vi "credentialCheck.vi"(0 "connection ID in":refnum<k5>, 1 "error in":errorcluster) -> (2 "connection ID out":refnum<k5>, 3 "user":string, 4 "error out":errorcluster)   [LabVIEW 2011]
panel:
  out "Error Parm":errorcluster
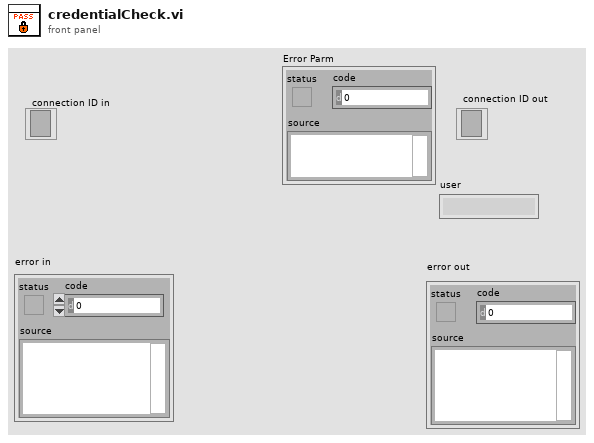
[diagram p1: front panel]
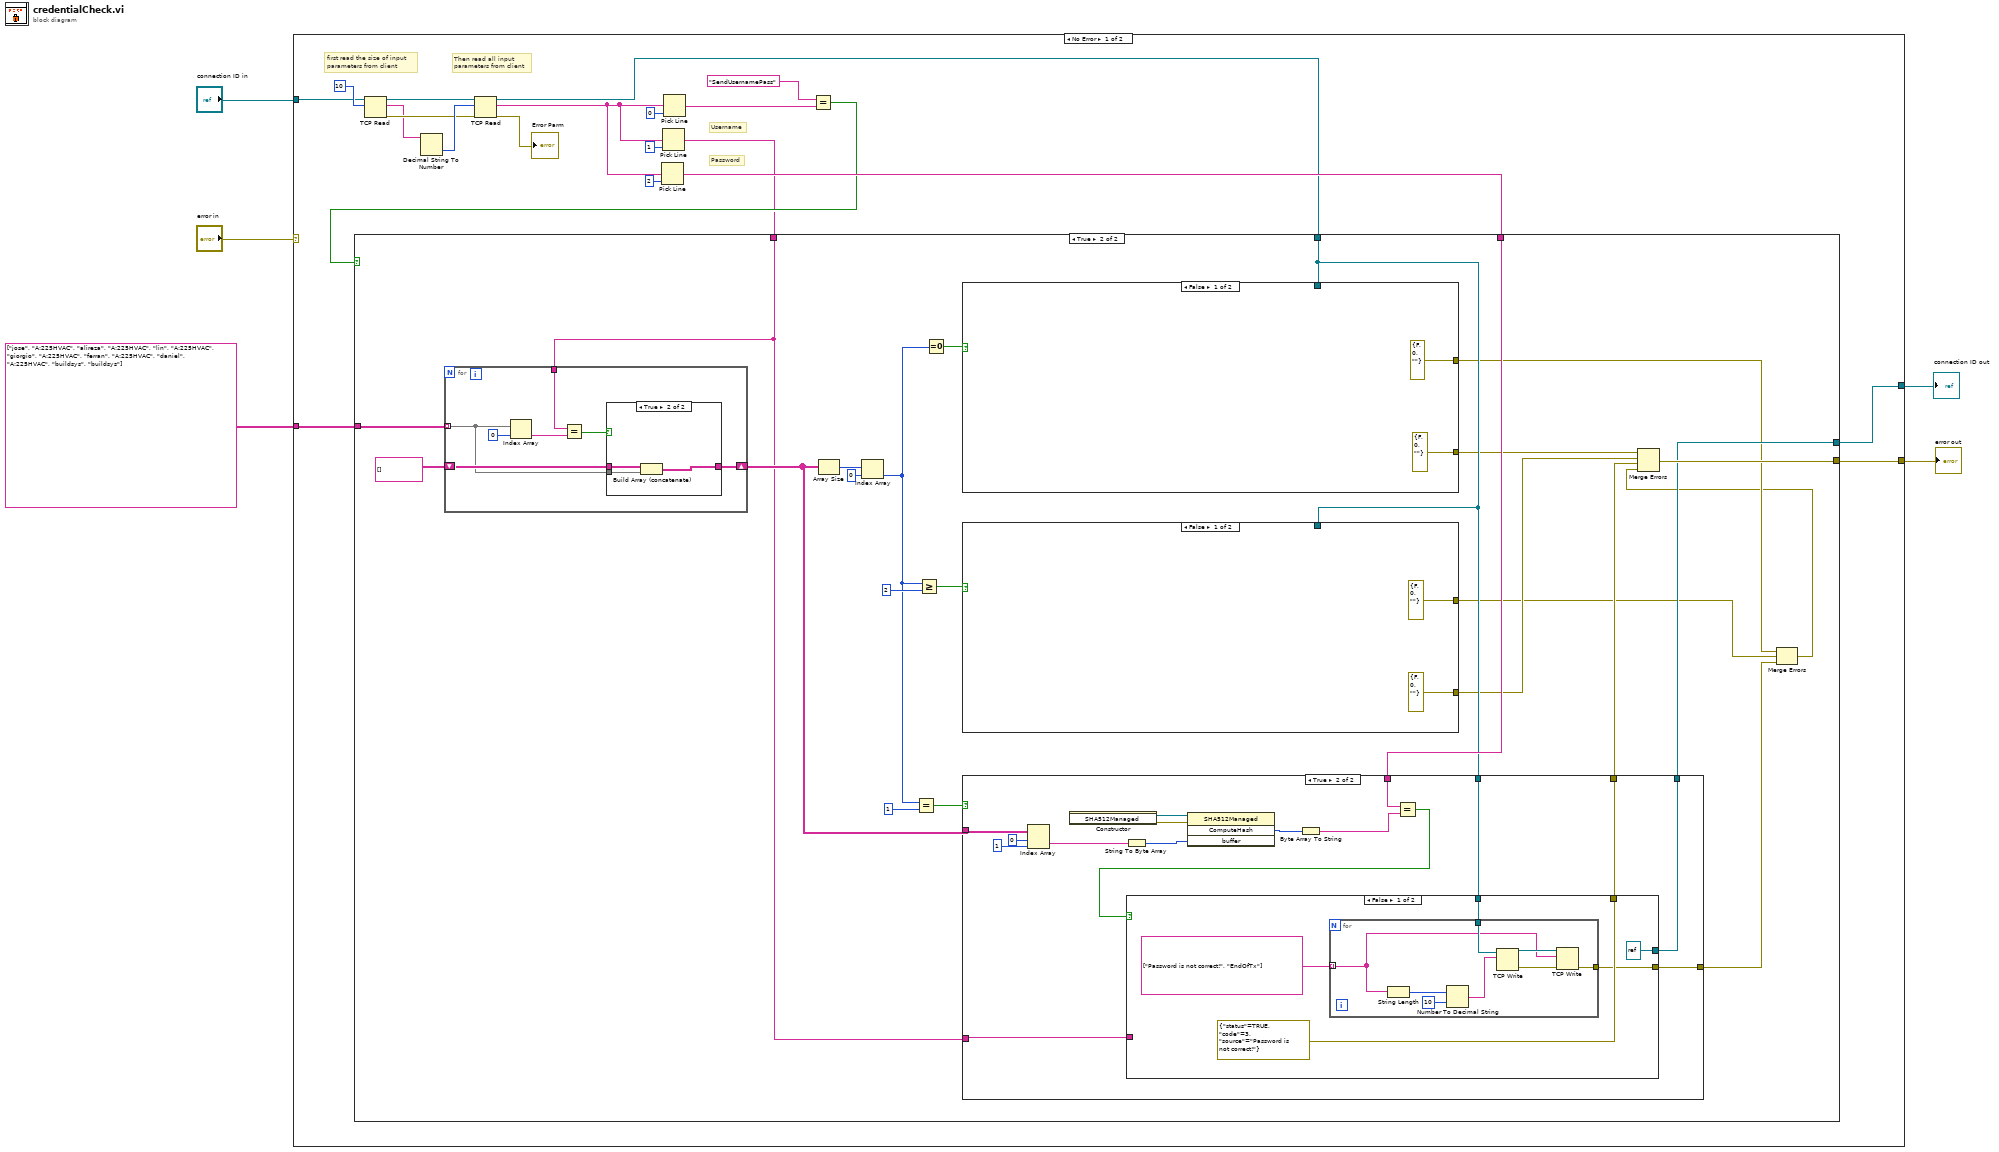
[diagram p0: block diagram]
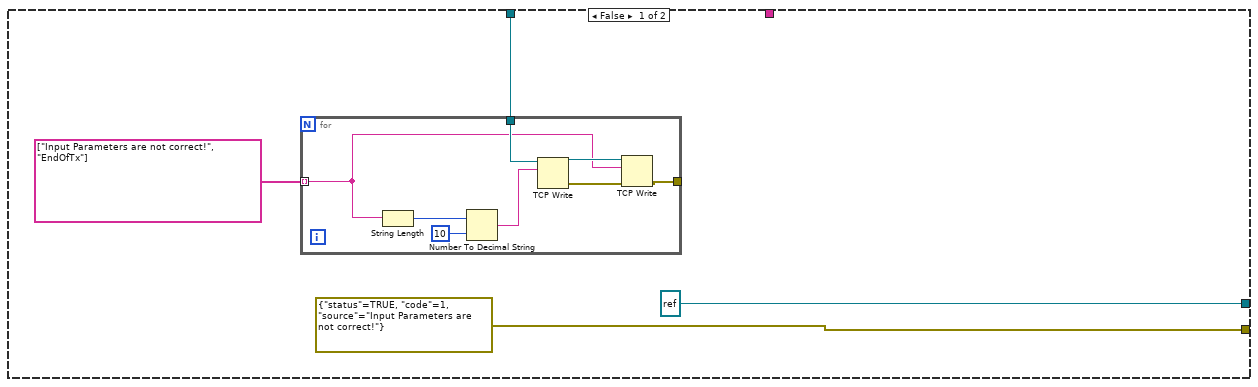
[diagram p2: hidden frame]
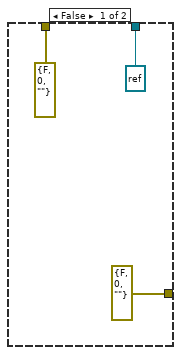
[diagram p3: hidden frame]
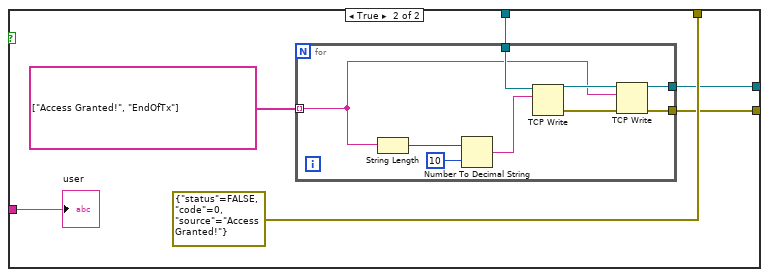
[diagram p4: hidden frame]
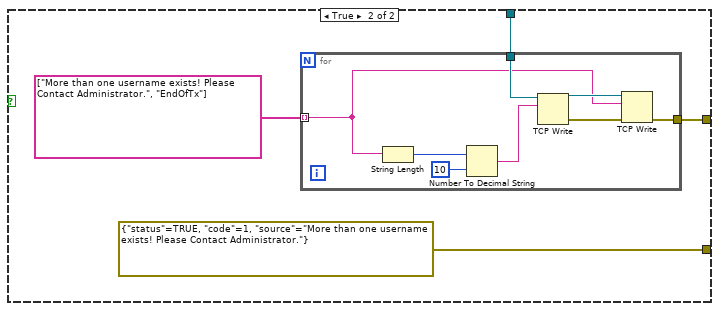
[diagram p5: hidden frame]
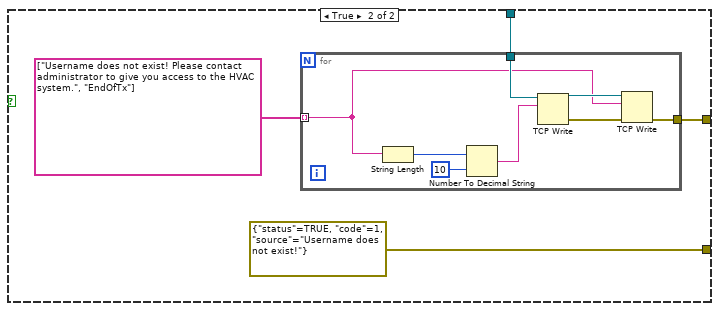
[diagram p6: hidden frame]
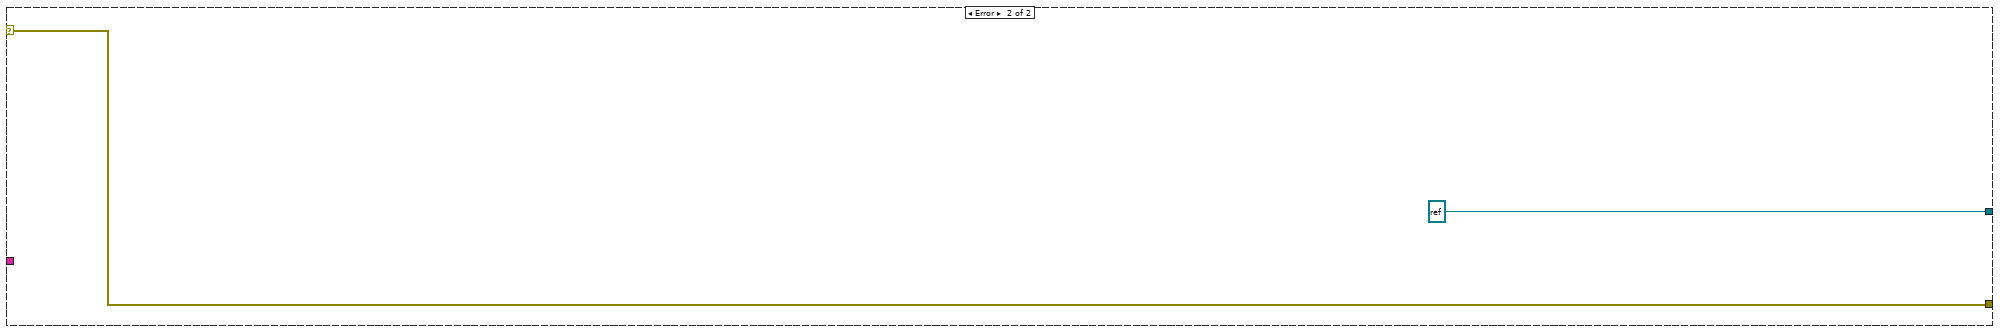
[diagram p8: hidden frame]
diagram:
  n1 = case shown="No Error" "error in" {
    selector: "error in" -> [_ w148]
    tunnel: "connection ID in" -> [w14 _]
    tunnel: [w10 refnum<k5> refnum ("connection ID in")] -> w5
    tunnel: [w11 w148] -> w2
    tunnel: string[][] [["jose", "A:225HVAC"], ["alireza", "A:225HVAC"], ["lin", "A:225HVAC"], ["giorgio", "A:225HVAC"], ["ferran", "A:225HVAC"], ["daniel", "A:225HVAC"], ["buildsys", "buildsys"]] -> [w9 _]
    frame No Error {
      # "Then read all input \nparameters from client"
      # "Password"
      # "Username"
      # "first read the size of input \nparameters from client"
      n2 = TCP Read(connection ID=w14, bytes to read=10) -> (connection ID out=w21:refnum<k5>, data out=w20:string, error out=w22:errorcluster)  [unwired: 3 in]
      n3 = Decimal String To Number(string=w20) -> (number=w23:i32)  [unwired: 2 in, 1 out]
      n4 = TCP Read(connection ID=w21, bytes to read=w23, error in (no error)=w22) -> (connection ID out=w7:refnum<k5>, data out=w25:string, error out=→"Error Parm":errorcluster)  [unwired: 2 in]
      n5 = Pick Line(multi-line string=w25, line index=2) -> (output string=w13:string)  [unwired: 1 in]
      n6 = Pick Line(multi-line string=w25, line index=1) -> (output string=w8:string)  [unwired: 1 in]
      n7 = Pick Line(multi-line string=w25, line index=0) -> (output string=w24:string)  [unwired: 1 in]
      n8 = Equal?(x="SendUsernamePass", y=w24) -> (x = y?=w12:bool)
      n9 = case shown="True" w12 {
        tunnel: w13 -> [_ w49]
        tunnel: [errorcluster {"status"=TRUE, "code"=1, "source"="Input Parameters are not correct!"} ("error out") w44] -> w11
        tunnel: [refnum<k5> refnum ("connection ID in") w43] -> w10
        tunnel: w9 -> [_ w59]
        tunnel: w8 -> [_ w42]
        tunnel: w7 -> [w26 w48]
        frame False {
          n10 = for {
            tunnel: w26 -> [w37]
            tunnel: string[] ["Input Parameters are not correct!", "EndOfTx"] -> [w31] mode=indexing
            tunnel: [w30] -> _
            n11 = String Length(string=w31) -> (length=w35:i32)
            n12 = Number To Decimal String(number=w35, width (-)=i16 10) -> (decimal integer string=w34:string)
            n13 = TCP Write(connection ID=w37, data in=w34) -> (connection ID out=w32:refnum<k5>, error out=w33:errorcluster)  [unwired: 2 in, 1 out]
            n14 = TCP Write(connection ID=w32, data in=w31, error in (no error)=w33) -> (error out=w30:errorcluster)  [unwired: 1 in, 2 out]
          }
        }
        frame True {
          n15 = for {
            shift-right: [w136] -> w50
            shift-left: string[][] [] -> [w138]
            tunnel: w59 -> [w137] mode=indexing
            tunnel: w42 -> [w140]
            n16 = Index Array(array=w137, index=0) -> (element=w141:string)
            n17 = Equal?(x=w140, y=w141) -> (x = y?=w139:bool)
            n18 = case shown="True" w139 {
              tunnel: w138 -> [w143 w146]
              tunnel: w137 -> [_ w145]
              tunnel: [w143 w144] -> w136
              frame False {
              }
              frame True {
                n19 = Build Array (concatenate)(w146, w145) -> (w144:string[][])
              }
            }
          }
          n20 = Array Size(array=w50) -> (size(s)=w58:i32[])
          n21 = Index Array(array=w58, index=0) -> (element=w52:i32)
          n22 = Equal?(x=w52, y=1) -> (x = y?=w53:bool)
          n23 = Greater Or Equal?(x=w52, y=2) -> (x >= y?=w54:bool)
          n24 = Equal To 0?(x=w52) -> (x = 0?=w56:bool)
          n25 = case shown="False" w56 {
            tunnel: w48 -> [_ w126]
            tunnel: [errorcluster {"status"=FALSE, "code"=0, "source"=""} ("error out") errorcluster {"status"=TRUE, "code"=1, "source"="Username does not exist!"} ("error out")] -> w47
            tunnel: [errorcluster {"status"=FALSE, "code"=0, "source"=""} ("error out") w124] -> w39
            frame False {
            }
            frame True {
              n26 = for {
                tunnel: w126 -> [w135]
                tunnel: string[] ["Username does not exist! Please contact administrator to give you access to the HVAC system.", "EndOfTx"] -> [w129] mode=indexing
                tunnel: [w128] -> w124
                n27 = String Length(string=w129) -> (length=w133:i32)
                n28 = Number To Decimal String(number=w133, width (-)=i16 10) -> (decimal integer string=w132:string)
                n29 = TCP Write(connection ID=w135, data in=w132) -> (connection ID out=w130:refnum<k5>, error out=w131:errorcluster)  [unwired: 2 in, 1 out]
                n30 = TCP Write(connection ID=w130, data in=w129, error in (no error)=w131) -> (error out=w128:errorcluster)  [unwired: 1 in, 2 out]
              }
            }
          }
          n31 = case shown="False" w54 {
            tunnel: w48 -> [_ w112]
            tunnel: [errorcluster {"status"=FALSE, "code"=0, "source"=""} ("error out") errorcluster {"status"=TRUE, "code"=1, "source"="More than one username exists! Please Contact Administrator."} ("error out")] -> w46
            tunnel: [errorcluster {"status"=FALSE, "code"=0, "source"=""} ("error out") w110] -> w40
            frame False {
            }
            frame True {
              n32 = for {
                tunnel: w112 -> [w121]
                tunnel: string[] ["More than one username exists! Please Contact Administrator.", "EndOfTx"] -> [w115] mode=indexing
                tunnel: [w114] -> w110
                n33 = String Length(string=w115) -> (length=w119:i32)
                n34 = Number To Decimal String(number=w119, width (-)=i16 10) -> (decimal integer string=w118:string)
                n35 = TCP Write(connection ID=w121, data in=w118) -> (connection ID out=w116:refnum<k5>, error out=w117:errorcluster)  [unwired: 2 in, 1 out]
                n36 = TCP Write(connection ID=w116, data in=w115, error in (no error)=w117) -> (error out=w114:errorcluster)  [unwired: 1 in, 2 out]
              }
            }
          }
          n37 = case shown="True" w53 {
            tunnel: w50 -> [_ w72]
            tunnel: w49 -> [_ w69]
            tunnel: w48 -> [_ w68]
            tunnel: [errorcluster {"status"=FALSE, "code"=0, "source"=""} ("error out") w67] -> w45
            tunnel: [refnum<k5> refnum ("connection ID in") w66] -> w43
            tunnel: w42 -> [_ w65]
            tunnel: [errorcluster {"status"=FALSE, "code"=0, "source"=""} ("error out") w64] -> w41
            frame False {
            }
            frame True {
              n38 = Index Array(array=w72, index (row)=0 ("index"), index (col)=1 ("disabled index (col)")) -> (element=w70:string)
              n39 = constructor class="SHA512Managed"() -> (reference out=w77:refnum<k24>, error out=w76:errorcluster)  [unwired: 3 in, 1 out]
              n40 = String To Byte Array(string=w70) -> (unsigned byte array=w75:u8[])
              n41 = invoke class="SHA512Managed" method="ComputeHash"(reference=w77, error in=w76, "buffer"=w75) -> ("ComputeHash"=w74:u8[])  [unwired: 1 in, 3 out]
              n42 = Byte Array To String(unsigned byte array=w74) -> (string=w78:string)
              n43 = Equal?(x=w69, y=w78) -> (x = y?=w79:bool)
              n44 = case shown="False" w79 {
                tunnel: w68 -> [w84 w97]
                tunnel: [errorcluster {"status"=TRUE, "code"=3, "source"="Password is not correct!"} ("error out") errorcluster {"status"=FALSE, "code"=0, "source"="Access Granted!"} ("error out")] -> w67
                tunnel: [refnum<k5> refnum ("connection ID in") w95] -> w66
                tunnel: w65 -> [_ w94]
                tunnel: [w80 w93] -> w64
                frame False {
                  n45 = for {
                    tunnel: w84 -> [w92]
                    tunnel: string[] ["Password is not correct!", "EndOfTx"] -> [w86] mode=indexing
                    tunnel: [w85] -> w80
                    n46 = String Length(string=w86) -> (length=w90:i32)
                    n47 = Number To Decimal String(number=w90, width (-)=i16 10) -> (decimal integer string=w89:string)
                    n48 = TCP Write(connection ID=w92, data in=w89) -> (connection ID out=w87:refnum<k5>, error out=w88:errorcluster)  [unwired: 2 in, 1 out]
                    n49 = TCP Write(connection ID=w87, data in=w86, error in (no error)=w88) -> (error out=w85:errorcluster)  [unwired: 1 in, 2 out]
                  }
                }
                frame True {
                  n50 = for {
                    tunnel: w97 -> [w107]
                    tunnel: string[] ["Access Granted!", "EndOfTx"] -> [w101] mode=indexing
                    tunnel: [w100] -> w95
                    tunnel: [w99] -> w93
                    n51 = String Length(string=w101) -> (length=w105:i32)
                    n52 = Number To Decimal String(number=w105, width (-)=i16 10) -> (decimal integer string=w104:string)
                    n53 = TCP Write(connection ID=w107, data in=w104) -> (connection ID out=w102:refnum<k5>, error out=w103:errorcluster)  [unwired: 2 in, 1 out]
                    n54 = TCP Write(connection ID=w102, data in=w101, error in (no error)=w103) -> (connection ID out=w100:refnum<k5>, error out=w99:errorcluster)  [unwired: 1 in, 1 out]
                  }
                  "user" <- w94
                }
              }
            }
          }
          n55 = Merge Errors(w39, w40, w41) -> (w38:errorcluster)
          n56 = Merge Errors(w47, w46, w45, w38) -> (w44:errorcluster)
        }
      }
    }
    frame Error {
    }
  }
  "connection ID out" <- w5
  "error out" <- w2
